vi "Actor Teardown Core.vi"(7 "Actor in":refnum<class "Actor.lvclass">, 11 "Self Actor State in":refnum<class "Self Actor State.lvclass">) -> (2 "Teardown?":bool, 5 "Actor out":refnum<class "Actor.lvclass">)   [LabVIEW 2021, in "jettl.lvlib" / "Self Actor State.lvclass"]
uses:
  Self Actor State.lvclass
  Actor/Actor.lvclass
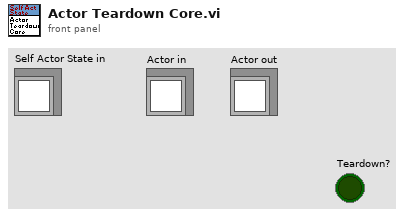
[diagram p1: front panel]
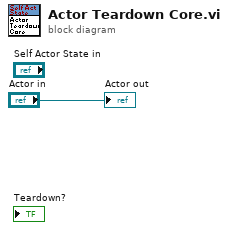
[diagram p0: block diagram]
diagram:
  "Actor out" <- "Actor in"
